vi "arreglosCluster.vi"() -> ()   [LabVIEW 2011]
uses:
  ControlArregloCluste.ctl
panel:
  out "Array":T1(array[cluster]) {"Temp 3" scale=0.0..60.0; "Temp 2" scale=0.0..60.0; "Temp1" scale=0.0..60.0}
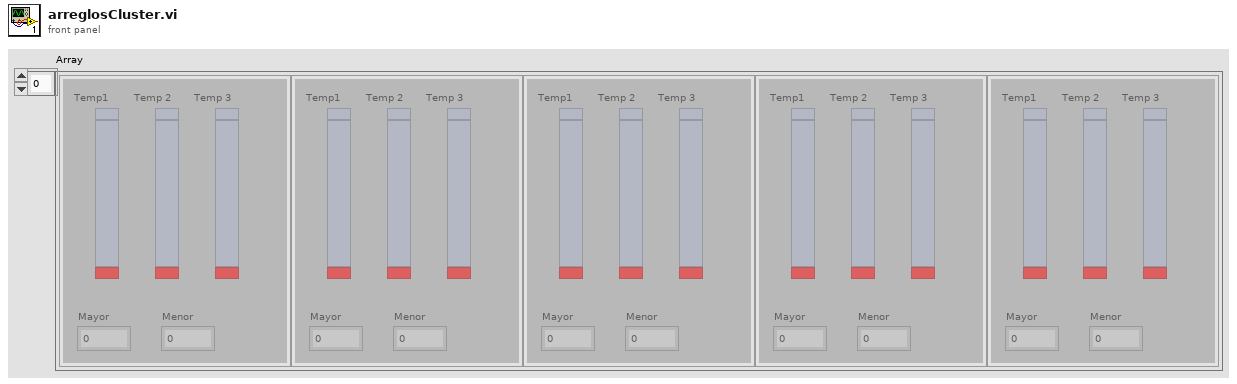
[diagram p1: front panel]
types:
  T1 = cluster{"Temp1":i32, "Temp 2":i32, "Temp 3":i32, "Mayor":dbl, "Menor":dbl}[]
  T2 = typedef "ControlArregloCluste.ctl" = enum16{"inicar arreglo", "ingresar Temperaturas", "obtener maximo y minimo", "finalizar"}
  T3 = cluster{"Temp1":i32, "Temp 2":i32, "Temp 3":i32, "Mayor":dbl, "Menor":dbl}
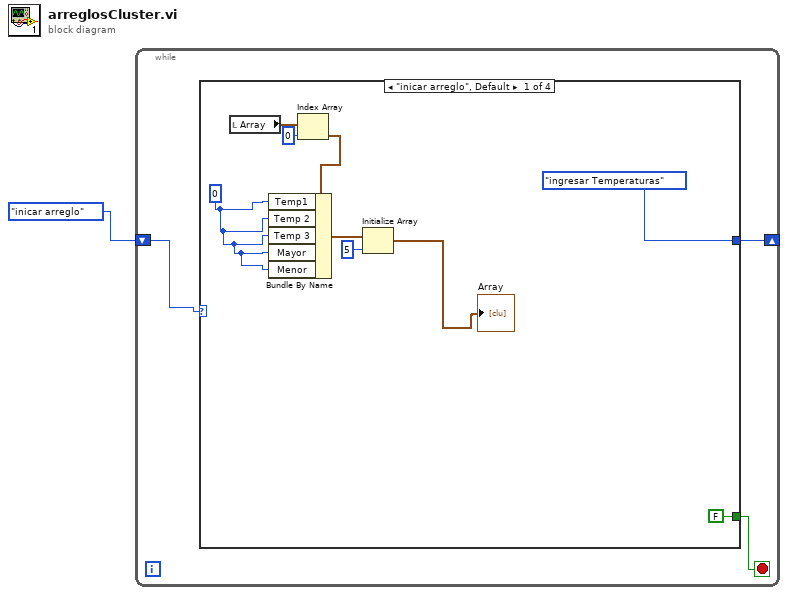
[diagram p0: block diagram]
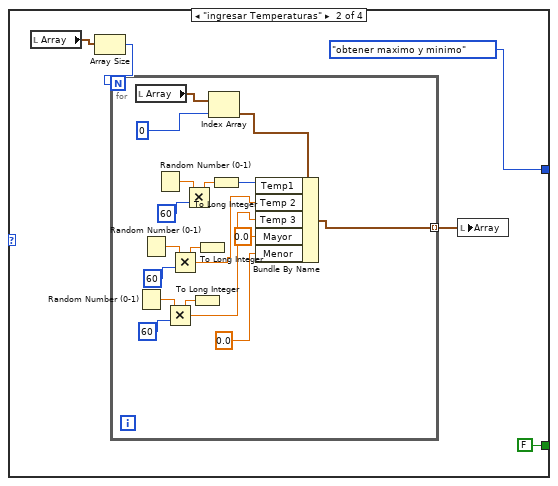
[diagram p2: hidden frame]
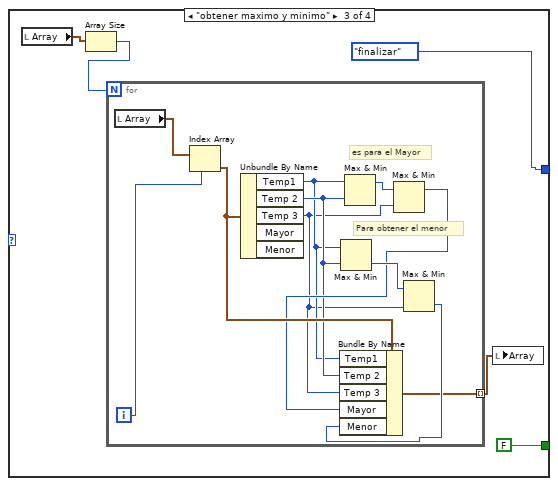
[diagram p3: hidden frame]
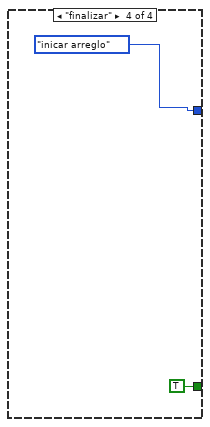
[diagram p4: hidden frame]
diagram:
  n1 = while {
    shift-right: [w3] -> _
    shift-left: ControlArregloCluste."inicar arreglo" -> [w4]
    stop <- w2 stop-if-true
    n2 = case shown="\"inicar arreglo\", Default" w4 {
      tunnel: [ControlArregloCluste."ingresar Temperaturas" ControlArregloCluste."obtener maximo y minimo" ControlArregloCluste."finalizar" ControlArregloCluste."inicar arreglo"] -> w3
      tunnel: [FALSE FALSE FALSE TRUE] -> w2
      frame "inicar arreglo", Default {
        w5 = 0
        n3 = local read "Array"() -> (w11:T1)
        n4 = Index Array "Index Array"(array=w11, index=0) -> (element=w9:T3)
        n5 = Bundle By Name(cluster=w9, "Temp1"=w5, "Temp 2"=w5, "Temp 3"=w5, "Mayor"=w5, "Menor"=w5) -> (w8:T3)
        n6 = Initialize Array "Initialize Array"(w8, 5 ("dimension size")) -> (→"Array":T1)
      }
      frame "ingresar Temperaturas" {
        n7 = local read "Array"() -> (w17:T1)
        n8 = Array Size(array=w17) -> (size(s)=w18:i32)
        n9 = for {
          N: w18 -> [_]
          tunnel: [w19] -> w16 mode=indexing
          n10 = local read "Array"() -> (w34:T1)
          n11 = Random Number (0-1)() -> (number: 0 to 1=w24:dbl)
          n12 = Random Number (0-1)() -> (number: 0 to 1=w27:dbl)
          n13 = Random Number (0-1)() -> (number: 0 to 1=w28:dbl)
          n14 = Multiply(x=w24, y=60) -> (x*y=w22:dbl)
          n15 = Multiply(x=w27, y=60) -> (x*y=w23:dbl)
          n16 = Multiply(x=w28, y=60) -> (x*y=w31:dbl)
          n17 = To Long Integer(number=w22) -> ()  [unwired: 1 out]
          n18 = To Long Integer(number=w23) -> ()  [unwired: 1 out]
          n19 = Index Array "Index Array"(array=w34, index=0) -> (element=w32:T3)
          n20 = To Long Integer(number=w31) -> (32bit integer=w30:i32)
          n21 = Bundle By Name "Bundle By Name"(cluster=w32, "Temp1"=w30, "Temp 2"=w23, "Temp 3"=w22, "Mayor"=0.0, "Menor"=0.0 ("Mayor")) -> (w19:T3)
        }
        n22 = local write "Array"(w16) -> ()
      }
      frame "obtener maximo y minimo" {
        n23 = local read "Array"() -> (w39:T1)
        n24 = Array Size(array=w39) -> (size(s)=w38:i32)
        n25 = for {
          N: w38 -> [_]
          tunnel: [w40] -> w37 mode=indexing
          i -> [w49]
          # "Para obtener el menor"
          # "es para el Mayor"
          n26 = local read "Array"() -> (w50:T1)
          n27 = Index Array "Index Array"(array=w50, index=w49) -> (element=w46:T3)
          n28 = Unbundle By Name "Unbundle By Name"(w46) -> ("Temp1"=w42:i32, "Temp 2"=w43:i32, "Temp 3"=w41:i32)  [unwired: 2 out]
          n29 = Max & Min(x=w42, y=w43) -> (min(x,y)=w47:i32)  [unwired: 1 out]
          n30 = Max & Min(x=w42, y=w43) -> (max(x,y)=w48:i32)  [unwired: 1 out]
          n31 = Max & Min(x=w48, y=w41) -> (max(x,y)=w45:i32)  [unwired: 1 out]
          n32 = Max & Min(x=w47, y=w41) -> (min(x,y)=w44:i32)  [unwired: 1 out]
          n33 = Bundle By Name(cluster=w46, "Temp1"=w42, "Temp 2"=w43, "Temp 3"=w41, "Mayor"=w45, "Menor"=w44) -> (w40:T3)
        }
        n34 = local write "Array"(w37) -> ()
      }
      frame "finalizar" {
      }
    }
  }
